vi "test-TimeInterpPose-ALL-TESTS.vi"(8 "error in (no error)":errorcluster) -> (0 "error out":errorcluster, 3 "All Passed":bool)   [LabVIEW 2019]
panel:
  out "Test 1":bool
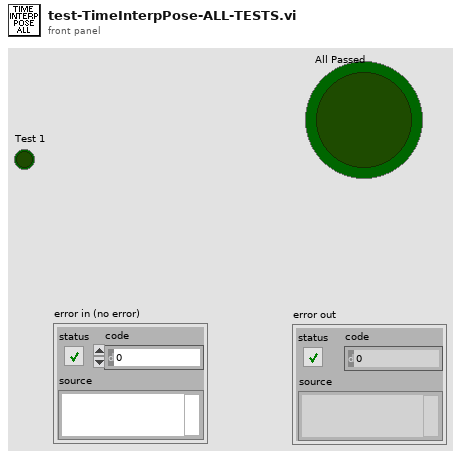
[diagram p1: front panel]
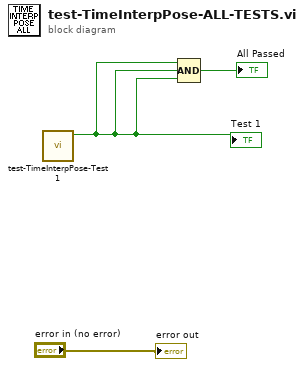
[diagram p0: block diagram]
diagram:
  n1 = call "test-TimeInterpPose-Test1.vi"() -> ("All tests passed"=w1:bool)  [unwired: 11 in]
  "Test 1" <- w1
  n2 = Compound Arithmetic op=AND(w1, w1, w1) -> (→"All Passed":bool)
  "error out" <- "error in (no error)"
